vi "SubVI_Acc_Filter.vi"(8 "에러 입력(에러 없음)":errorcluster, 10 "Acc Index":i32, 11 "Raw Data":dbl[][](array[numeric])) -> (0 "에러 출력":errorcluster, 3 "Acc. Filltered Raw Data":dbl[][](array[numeric]))   [LabVIEW 2013]
uses:
  <vilib>/Analysis/3filter.llb/Bessel Filter (DBL).vi
  <vilib>/Analysis/NI_AALBase.lvlib
panel:
  out "웨이브폼 그래프 4":dbl[][](graph)
  out "웨이브폼 그래프 3":dbl[][](graph)
  out "웨이브폼 그래프 2":dbl[](graph)
  out "웨이브폼 그래프":dbl[](graph)
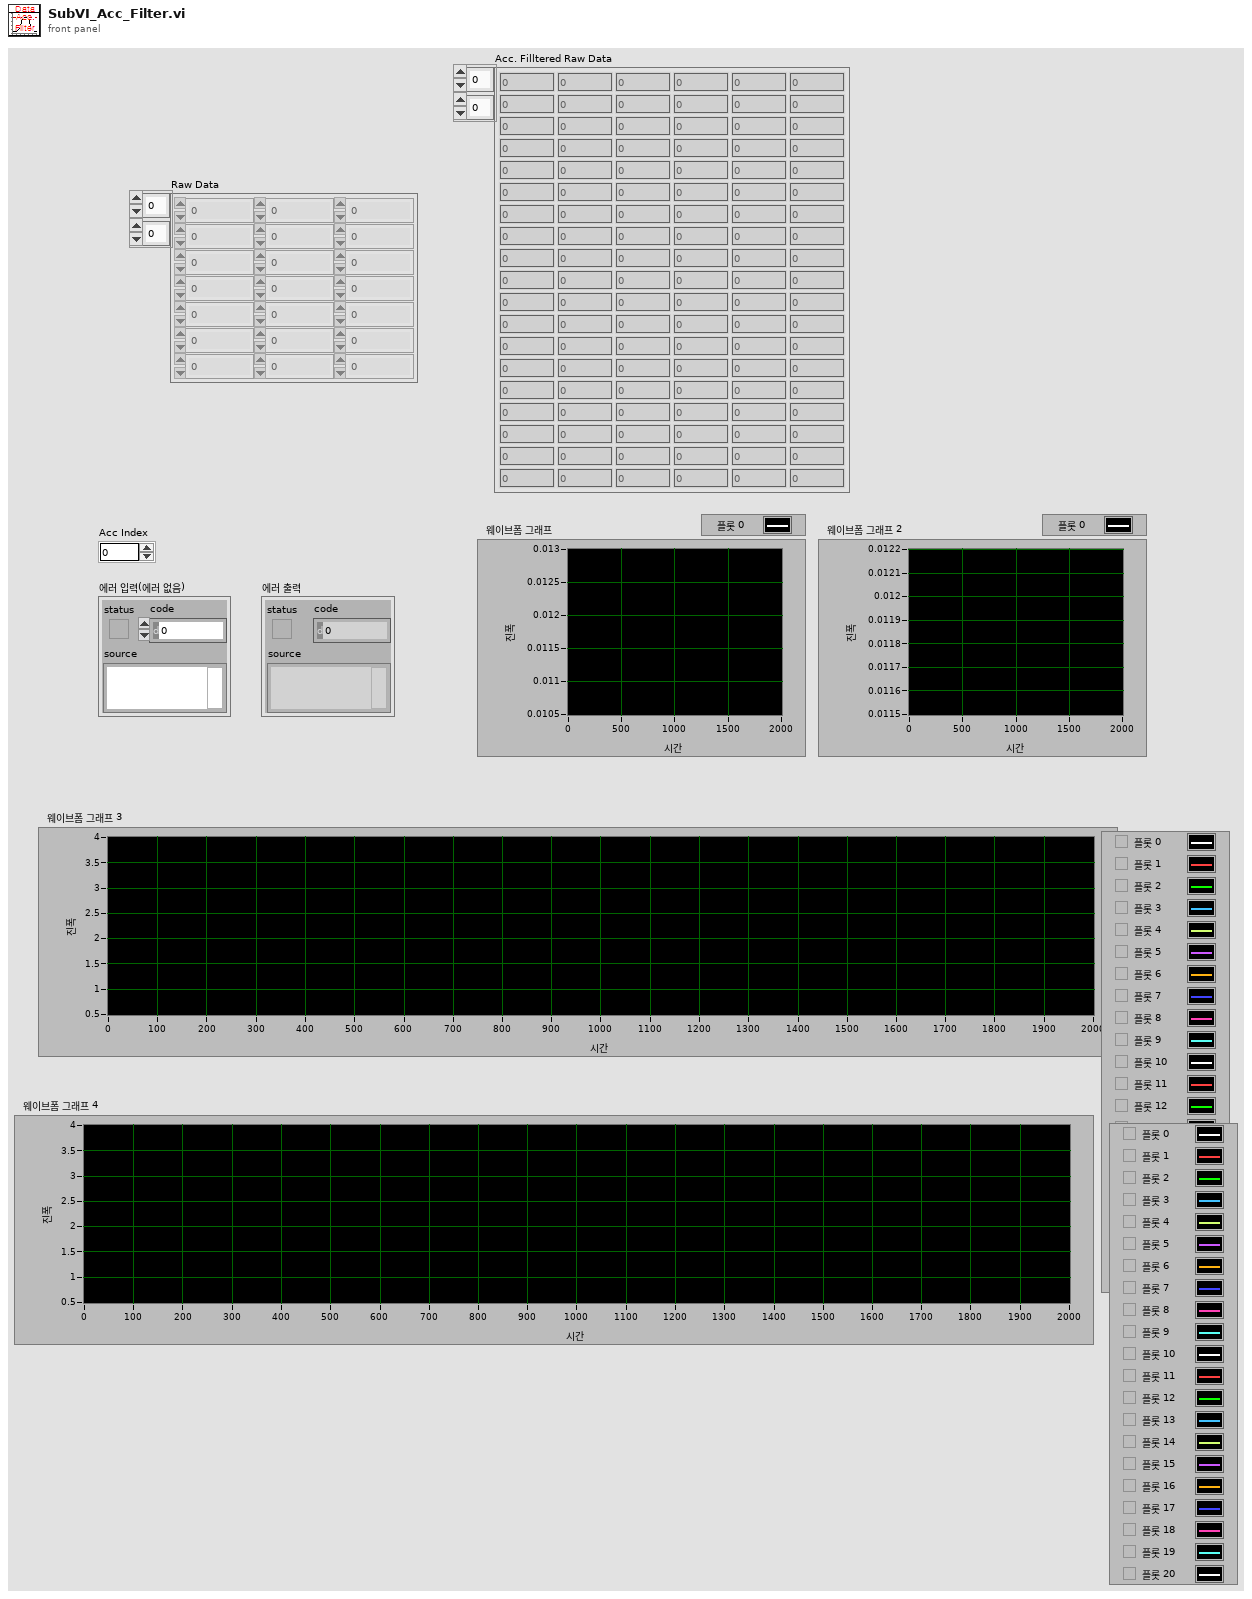
[diagram p1: front panel]
types:
  T1 = enum32{"Lowpass", "Highpass", "Bandpass", "Bandstop"}
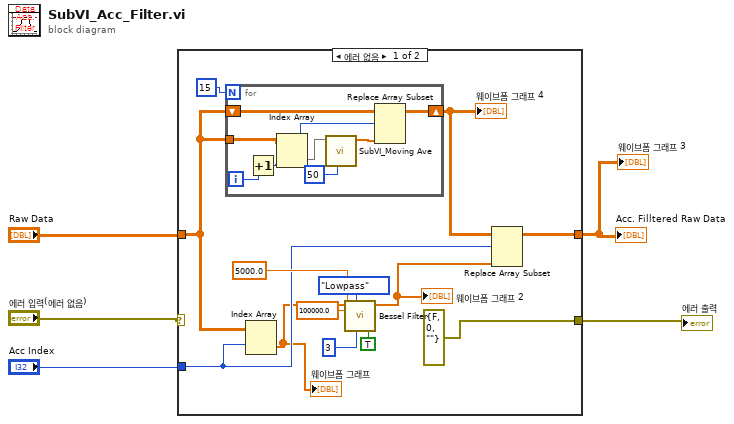
[diagram p0: block diagram]
diagram:
  n1 = case shown="에러 없음" "에러 입력(에러 없음)" {
    selector: "에러 입력(에러 없음)" -> [_ w28]
    tunnel: "Acc Index" -> [w12 _]
    tunnel: "Raw Data" -> [w7 w27]
    tunnel: [errorcluster {"status"=FALSE, "code"=0, "source"=""} ("error IO") w28] -> w4
    tunnel: [w11 w27] -> w1
    frame No Error {
      n2 = for {
        N: 15 -> [_]
        tunnel: w7 -> [w24]
        shift-right: [w19] -> w6
        shift-left: w7 -> [w22]
        i -> [w25]
        n3 = Increment(x=w25) -> (x+1=w20:i32)
        n4 = Index Array(array=w24, index (row)=w20) -> (element=w23:dbl[])  [unwired: 1 in]
        n5 = call "SubVI_Moving Ave.vi"("Ave. NO"=50, "Data"=w23) -> ("Filtered Data"=w21:dbl[])  [unwired: 9 in]
        n6 = Replace Array Subset(array=w22, new element=w21, index (row)=w20) -> (w19:dbl[][])  [unwired: 1 in]
      }
      "웨이브폼 그래프 4" <- w6
      n7 = Index Array(array=w7, index (row)=w12) -> (element=w10:dbl[])  [unwired: 1 in]
      "웨이브폼 그래프" <- w10
      n8 = call-poly <vilib>:"Bessel Filter.vi"("init/cont (init:F)"=TRUE, "order"=3, "filter type"=T1."Lowpass", "low cutoff freq: fl"=5000.0, "sampling freq: fs"=100000.0, "X"=w10) -> ("Filtered X"=w9:dbl[])  [unwired: 2 in, 1 out]
      "웨이브폼 그래프 2" <- w9
      n9 = Replace Array Subset(array=w6, new element=w9, index (row)=w12) -> (w11:dbl[][])  [unwired: 1 in]
    }
    frame Error {
    }
  }
  "에러 출력" <- w4
  "Acc. Filltered Raw Data" <- w1
  "웨이브폼 그래프 3" <- w1
